vi "rsscope Instrument Options.vi"(0 "VISA resource name":refnum<visa-resource-name>, 11 "error in (no error)":errorcluster) -> (4 "VISA resource name out":refnum<visa-resource-name>, 6 "Instrument Version":string, 10 "Options List":string, 14 "Inst Ver Index":i32, 15 "error out":errorcluster)   [LabVIEW 2018]
doc: "This VI returns the instrument version number and the list of options which the instrument is equipped with.\n\nRemote-control commands:\n*IDN?\n*OPT?"
uses:
  _utility/rsscope_core_global.vi
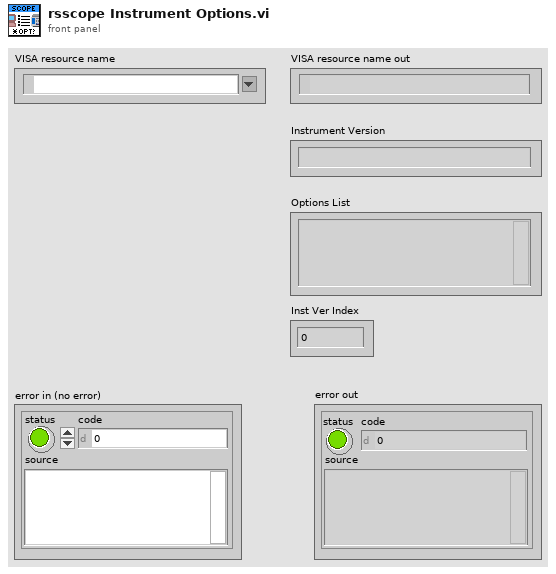
[diagram p1: front panel]
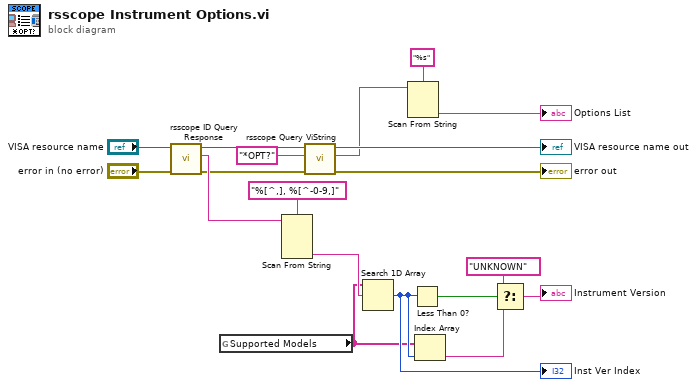
[diagram p0: block diagram]
diagram:
  n1 = call "rsscope ID Query Response.vi"("error in (no error)"="error in (no error)", "VISA resource name"="VISA resource name") -> ("error out"=w5:errorcluster, "ID Query Response"=w8:string, "VISA resource name out"=w4:refnum<visa-resource-name>)  [unwired: 7 in]
  n2 = global read "rsscope_core_global.vi" "Supported Models"() -> (w9:string[])
  n3 = Scan From String(format string="%[^,], %[^-0-9,]", input string=w8) -> (output 2=w12:string)  [unwired: 5 in, 3 out]
  n4 = call "rsscope Query ViString.vi"("error in (no error)"=w5, "Query"="*OPT?", "VISA resource name"=w4) -> ("error out"=→"error out":errorcluster, "Response Value"=w1:string, "VISA resource name out"=→"VISA resource name out":refnum<visa-resource-name>)  [unwired: 6 in]
  n5 = Search 1D Array(1D array=w9, element=w12) -> (index of element=w10:i32)  [unwired: 1 in]
  "Inst Ver Index" <- w10
  n6 = Scan From String(format string="%s", input string=w1) -> (output 1=→"Options List":string)  [unwired: 3 in, 3 out]
  n7 = Less Than 0?(x=w10) -> (x < 0?=w15:bool)
  n8 = Index Array(array=w9, index=w10) -> (element=w14:string)
  n9 = Select(t="UNKNOWN", s=w15, f=w14) -> (s? t:f=→"Instrument Version":string)
